vi "Apply Deviation.vi"(8 "error in (no error)":errorcluster, 11 "Tool Path in":refnum<class "Tool Path.lvclass">) -> (0 "error out":errorcluster, 3 "Tool Path out":refnum<class "Tool Path.lvclass">)   [LabVIEW 2019, in "Tool Path.lvclass"]
uses:
  Tool Path.lvclass
  subVIs/typedefs/Schedule Types/Schedule--Formula.ctl
  Settings/Path Settings/Path Settings.lvclass/Path Settings.ctl
  Settings/Path Settings/Path Settings.lvclass
  Settings/ObjectSettings/ObjectSettings.lvclass
  <vilib>/gmath/NI_Gmath.lvlib
  Tool Object/Tool Object.lvclass
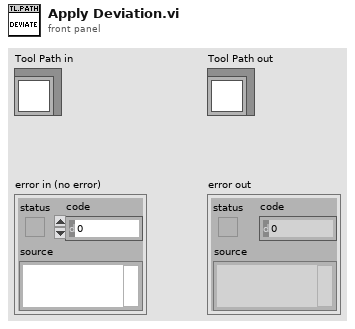
[diagram p1: front panel]
types:
  T1 = typedef "Schedule--Formula.ctl" = cluster{"formula":string, "formula length (nm)":dbl, "formula resolution (nm)":dbl}
  T2 = typedef "PathCommands.lvclass/Point.ctl" = cluster{"X":dbl, "Y":dbl}
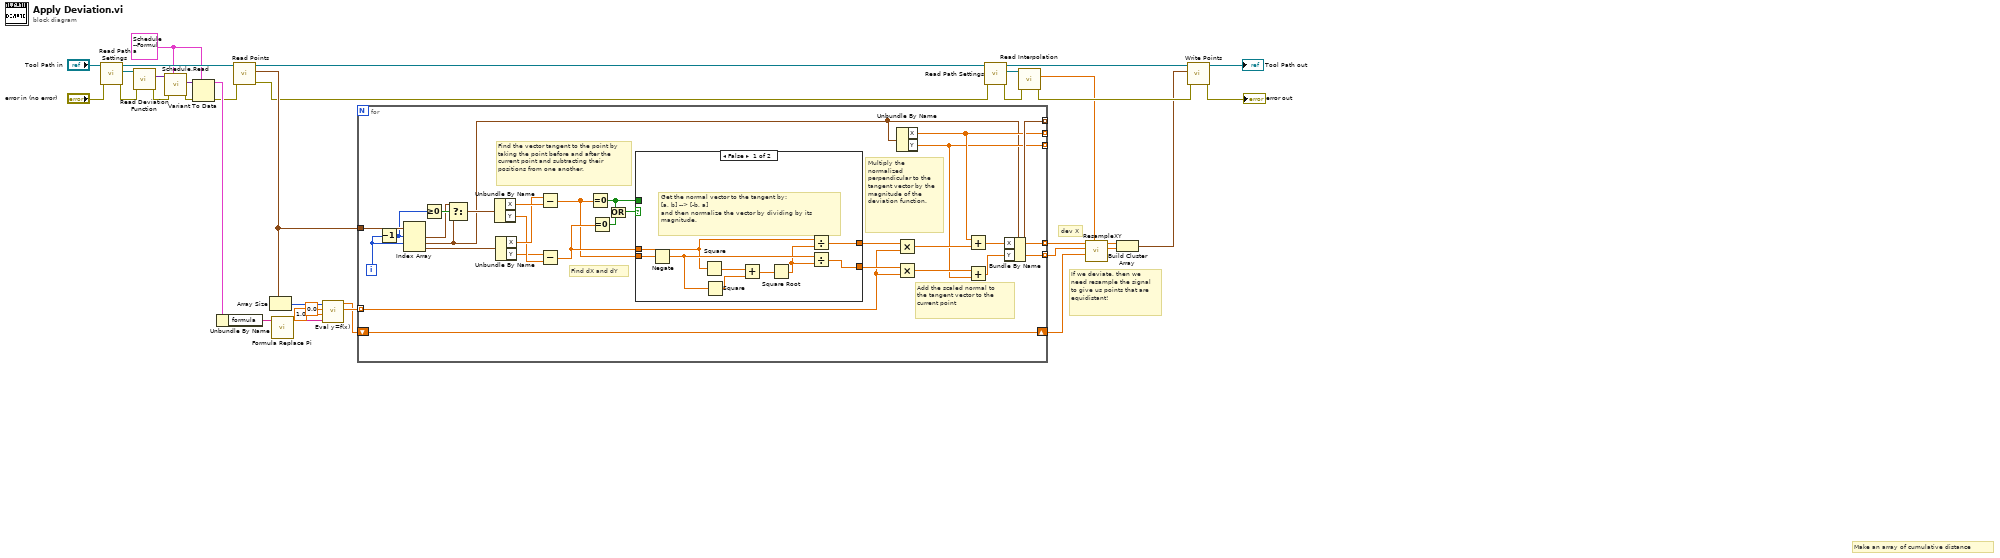
[diagram p0: block diagram]
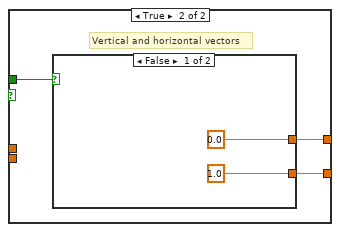
[diagram p2: hidden frame]
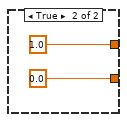
[diagram p3: hidden frame]
diagram:
  w24 = T1 {"formula"="1*(step(170-t)*cos(0.62831853071*t)+step(t-170)*cos(0.62831853071*(t-170))*(-1))", "formula length (nm)"=340.0, "formula resolution (nm)"=0.001} ("Formula")
  # "If we deviate, then we need resample the signal to give us points that are equidistant!"
  # "dev X"
  # "Make an array of cumulative distance"
  n1 = call-dynamic "Read Path Settings.vi"("error in (no error)"="error in (no error)", "Tool Path in"="Tool Path in") -> ("error out"=w23:errorcluster, "Path Settings.lvclass"=w34:refnum<class "Path Settings.lvclass">, "Tool Path out"=w28:refnum<class "Tool Path.lvclass">)  [unwired: 7 in]
  n2 = call-dynamic "Read Deviation Function.vi"("error in (no error)"=w23, "Path Settings in"=w34) -> ("error out"=w10:errorcluster, "Deviation Function"=w31:variant)  [unwired: 7 in, 1 out]
  n3 = call "Schedule.Read.vi"("Data to Read"=w24, "error in (no error)"=w10, "LUT In"=w31) -> ("error out"=w30:errorcluster, "Data Out"=w33:variant)  [unwired: 6 in, 1 out]
  n4 = Variant To Data(error in=w30, type=w24, Variant=w33) -> (data=w32:T1, error out=w22:errorcluster)
  n5 = Unbundle By Name(w32) -> ("formula"=w2:string)
  n6 = call-dynamic "Read Points.vi"("error in (no error)"=w22, "Tool Object in"=w28) -> ("error out"=w11:errorcluster, "Points"=w17:T2[], "Tool Object out"=w12:refnum<class "Tool Path.lvclass">)  [unwired: 7 in]
  n7 = Array Size(array=w17) -> (size(s)=w19:i32)
  n8 = call "Formula Replace Pi.vi"("Formula In"=w2) -> ("Formula Out"=w1:string)  [unwired: 4 in]
  n9 = call <vilib>:"Eval y=f(x).vi"("formula"=w1, "end"=1.0, "start"=0.0, "number of points"=w19) -> ("Y Values"=w25:dbl[], "X Values"=w18:dbl[])  [unwired: 2 out]
  n10 = for {
    tunnel: w17 -> [w63]
    tunnel: w25 -> [w47] mode=indexing
    tunnel: [w46] -> _ mode=indexing
    tunnel: [w45] -> w8 mode=indexing
    tunnel: [w44] -> w9 mode=indexing
    tunnel: [w43] -> _ mode=indexing
    tunnel: [w42] -> _ mode=indexing
    shift-right: [w36] -> w7
    shift-left: w18 -> [w36]
    i -> [w52]
    # "Add the scaled normal to the tangent vector to the current point"
    # "Multiply the normalized perpendicular to the tangent vector by the magnitude of the deviation function."
    # "Find the vector tangent to the point by taking the point before and after the current point and subtracting their positions from one another."
    # "Find dX and dY"
    n11 = Decrement(x=w52) -> (x-1=w41:i32)
    n12 = Index Array(array=w63, index #1=w41, index #2=w52) -> (element #1=w37:T2, element #2=w38:T2, element #3=w62:T2)  [unwired: 1 in]
    n13 = Greater Or Equal To 0?(x=w41) -> (x >= 0?=w40:bool)
    n14 = Select(t=w37, s=w40, f=w38) -> (s? t:f=w39:T2)
    n15 = Unbundle By Name(w39) -> ("X"=w61:dbl, "Y"=w59:dbl)
    n16 = Unbundle By Name(w62) -> ("X"=w60:dbl, "Y"=w58:dbl)
    n17 = Subtract(x=w60, y=w61) -> (x-y=w50:dbl)
    n18 = Subtract(x=w58, y=w59) -> (x-y=w51:dbl)
    n19 = Equal To 0?(x=w50) -> (x = 0?=w53:bool)
    n20 = Equal To 0?(x=w51) -> (x = 0?=w54:bool)
    n21 = Or(x=w53, y=w54) -> (x .or. y?=w55:bool)
    n22 = case shown="False" w55 {
      tunnel: [w65 w73] -> w48
      tunnel: [w71 w74] -> w49
      tunnel: w50 -> [w72 _]
      tunnel: w51 -> [w64 _]
      tunnel: w53 -> [_ w75]
      frame False {
        # "Get the normal vector to the tangent by:\n[a, b] --> [-b, a]\nand then normalize the vector by dividing by its magnitude."
        n23 = Negate(x=w72) -> (-x=w67:dbl)
        n24 = Square(x=w64) -> (x^2=w70:dbl)
        n25 = Square(x=w67) -> (x^2=w69:dbl)
        n26 = Add(x=w70, y=w69) -> (x+y=w68:dbl)
        n27 = Square Root(x=w68) -> (sqrt(x)=w66:dbl)
        n28 = Divide(x=w64, y=w66) -> (x/y=w71:dbl)
        n29 = Divide(x=w67, y=w66) -> (x/y=w65:dbl)
      }
      frame True {
        # "Vertical and horizontal vectors"
        n30 = case shown="False" w75 {
          tunnel: [0.0 1.0] -> w74
          tunnel: [1.0 0.0] -> w73
          frame False {
          }
          frame True {
          }
        }
      }
    }
    n31 = Multiply(x=w49, y=w47) -> (x*y=w56:dbl)
    n32 = Multiply(x=w48, y=w47) -> (x*y=w57:dbl)
    n33 = Unbundle By Name(w38) -> ("X"=w43:dbl, "Y"=w42:dbl)
    n34 = Add(x=w43, y=w56) -> (x+y=w44:dbl)
    n35 = Add(x=w57, y=w42) -> (x+y=w45:dbl)
    n36 = Bundle By Name(cluster=w38, "X"=w44, "Y"=w45) -> (w46:T2)
  }
  n37 = call-dynamic "Read Path Settings.vi"("error in (no error)"=w11, "Tool Path in"=w12) -> ("error out"=w20:errorcluster, "Path Settings.lvclass"=w21:refnum<class "Path Settings.lvclass">, "Tool Path out"=w16:refnum<class "Tool Path.lvclass">)  [unwired: 7 in]
  n38 = call "Read Interpolation.vi"("error in (no error)"=w20, "Path Settings in"=w21) -> ("error out"=w14:errorcluster, "Interpolation"=w6:dbl)  [unwired: 7 in, 1 out]
  n39 = call "ResampleXY.vi"("Interpolation Distance"=w6, "t"=w7, "Y"=w8, "X"=w9) -> ("Resampled Y"=w4:dbl[], "Resampled X"=w5:dbl[])  [unwired: 5 in, 1 out]
  n40 = Build Cluster Array(w5, w4) -> (w3:cluster{"Numeric":dbl, "Numeric":dbl}[])
  n41 = call-dynamic "Write Points.vi"("error in (no error)"=w14, "Points"=w3, "Tool Object in"=w16) -> ("error out"=→"error out":errorcluster, "Tool Object out"=→"Tool Path out":refnum<class "Tool Path.lvclass">)  [unwired: 7 in]
